vi "Add Abstract Message to Actor.vi"(8 "error in (no error)":errorcluster, 9 "Abstract Message Path":path, 10 "Target Actor in":refnum<vi>) -> (0 "error out":errorcluster)   [LabVIEW 2020, in "Message Maker.lvlib"]
uses:
  Message Maker.lvlib
  <resource>/Framework/Providers/LVClassLibrary/NewAccessors/MemberVICreation.lvlib
  <vilib>/Utility/EditLVLibs/Edit LVLibs.lvlib
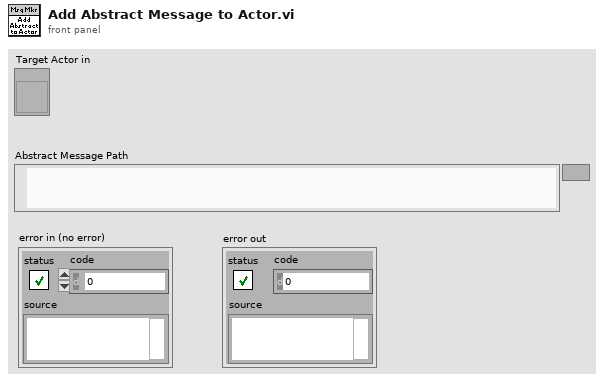
[diagram p1: front panel]
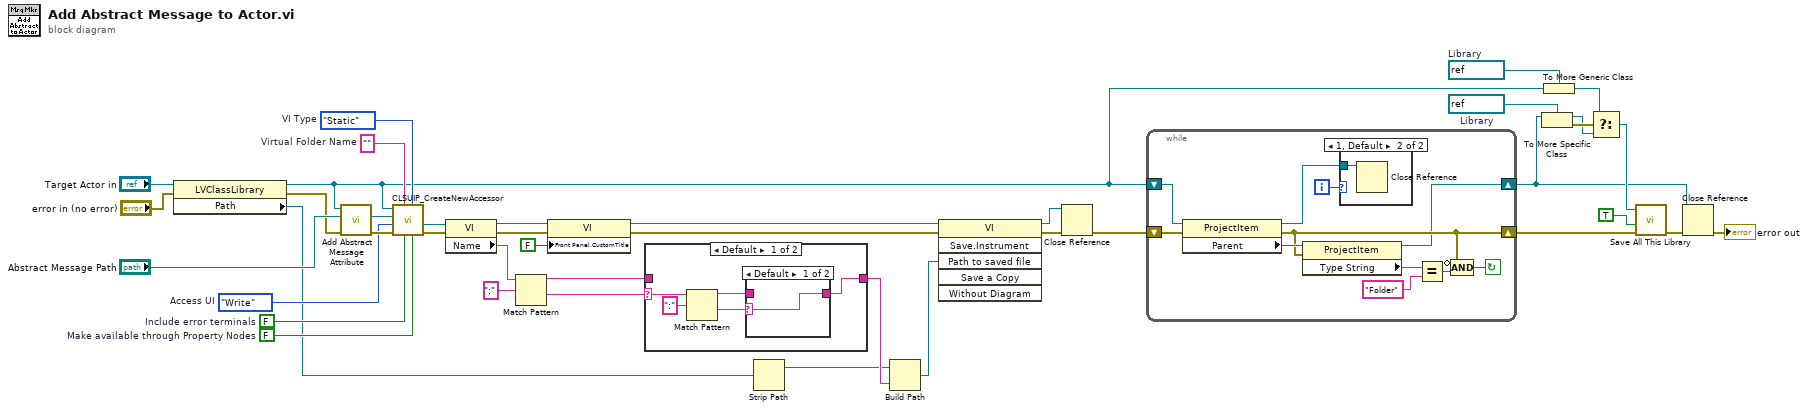
[diagram p0: block diagram]
diagram:
  w33 = ""  # Virtual Folder Name
  w34 = enum32{"Dynamic", "Static"}."Static"  # VI Type
  w32 = enum16{"Read", "Write", "R/W"}."Write"  # Access UI
  w35 = FALSE  # Make available through Property Nodes
  w36 = FALSE  # Include error terminals
  w37 = refnum<vi> refnum  # Library
  w38 = refnum<vi> refnum  # Library
  n1 = property class="LVClassLibrary"(reference="Target Actor in", error in="error in (no error)") -> (reference out=w4:refnum<vi>, error out=w17:errorcluster, "Path"=w16:path)
  n2 = call "Add Abstract Message Attribute.vi"("error in (no error)"=w17, "Abstract Message Path"="Abstract Message Path", "Target Actor in"=w4) -> ("error out"=w41:errorcluster, "Abstract Message Control"=w39:refnum<vi>)  [unwired: 7 in]
  n3 = call <resource>:"CLSUIP_CreateNewAccessor.vi"("Make available through Property Nodes"=w35, "VI Type"=w34, "Include error terminals"=w36, "Virtual Folder Name"=w33, "error in (no error)"=w41, "Access UI"=w32, "PDC Item Refnum"=w39, "LVClassLibrary Ref"=w4) -> ("error out"=w21:errorcluster, "Write VI"=w20:refnum<vi>)  [unwired: 1 in, 1 out]
  n4 = property class="VI"(reference=w20, error in=w21) -> (reference out=w8:refnum<vi>, error out=w30:errorcluster, "Name"=w25:string)
  n5 = Match Pattern(string=w25, regular expression=":") -> (before substring=w28:string, after substring=w27:string)  [unwired: 1 in, 2 out]
  n6 = property class="VI"(reference=w8, error in=w30, "Front Panel.CustomTitle"=FALSE ("Front Panel Window:Custom Title")) -> (reference out=w7:refnum<vi>, error out=w9:errorcluster)
  n7 = case shown="Default" w27 {
    selector: w27 -> [w45 _]
    tunnel: w28 -> [_ w49]
    tunnel: [w42 w49] -> w24
    frame Default {
      n8 = Match Pattern(string=w45, regular expression=":") -> (before substring=w43:string, after substring=w44:string)  [unwired: 1 in, 2 out]
      n9 = case shown="Default" w44 {
        selector: w44 -> [w47 _]
        tunnel: w43 -> [_ w48]
        tunnel: [w47 w48] -> w42
        frame Default {
        }
        frame "" {
        }
      }
    }
    frame "" {
    }
  }
  n10 = Strip Path(path=w16) -> (stripped path=w22:path)  [unwired: 1 out]
  n11 = Build Path(base path=w22, name or relative path=w24) -> (appended path=w23:path)
  n12 = invoke class="VI" method="Save.Instrument"(reference=w7, error in=w9, "Path to saved file"=w23) -> (reference out=w29:refnum<vi>, error out=w31:errorcluster)  [unwired: 3 in, 4 out]
  n13 = Close Reference(reference=w29, error in (no error)=w31) -> (error out=w3:errorcluster)
  n14 = while {
    shift-right: [w54] -> w2
    shift-left: w3 -> [w59]
    shift-right: [w50] -> w1
    shift-left: w4 -> [w60]
    i -> [w51]
    stop <- w53 continue-if-true
    n15 = property class="ProjectItem"(reference=w60, error in=w59) -> (reference out=w52:refnum<vi>, error out=w54:errorcluster, "Parent"=w58:refnum<vi>)
    n16 = property class="ProjectItem"(reference=w58, error in=w54) -> (reference out=w50:refnum<vi>, "Type String"=w57:string)  [unwired: 1 out]
    n17 = case shown="1, Default" w51 {
      tunnel: w52 -> [_ w61]
      frame 0 {
      }
      frame 1, Default {
        n18 = Close Reference(reference=w61) -> ()  [unwired: 1 in, 1 out]
      }
    }
    n19 = Equal?(x=w57, y="Folder") -> (x = y?=w55:bool)
    n20 = Compound Arithmetic op=AND(invert w54, w55) -> (w53:bool)
  }
  n21 = To More Specific Class(target class=w37, reference=w1) -> (specific class reference=w10:refnum<vi>, error out=w13:errorcluster)  [unwired: 1 in]
  n22 = To More Generic Class(target class=w38, reference=w4) -> (generic class reference=w11:refnum<vi>)
  n23 = Select(t=w11, s=w13, f=w10) -> (s? t:f=w12:refnum<vi>)
  n24 = call <vilib>:"Save All This Library.vi"("error in (no error)"=w2, "Save Only Modified VIs and Libraries? (F)"=TRUE, "Library in"=w12) -> ("error out"=w15:errorcluster)  [unwired: 7 in, 1 out]
  n25 = Close Reference(reference=w1, error in (no error)=w15) -> (error out=→"error out":errorcluster)
